vi "Robot Global Data.vi"() -> ()   [LabVIEW 2018]
doc: "This global VI can contain as many global variables as you need. Place a control on the panel, give it a good name. To read or write to it from a VI, drag the icon to the diagram of that VI. You can also drag from the project. Click on the node to change which global you access. You shouldn't have multiple locations writing to a global or it will cause a race-condition."
uses:
  <vilib>/Rock Robotics/WPI/DriverStation/WPI_DriverStationRobotMode2.ctl
panel:
  in  "Rottion_Control":dbl
  in  "Stage2_MotorControl 2":dbl
  in  "Stage1_MotorControl":dbl
  in  "manControl":bool
  out "DriverControllerButton12_input":bool
  in  "Stage 2_Lift PositionCurrent":string(combo)
  out "LIFT_EMERGENCY_STOP":bool
  in  "Lift Position_Desired":string(combo)
  out "DriverControllerButton11_input":bool
  out "DriveControllerButton10_input":bool
  out "DriveControllerButton9_input":bool
  out "DriveControllerButton8_input":bool
  out "DriveControllerButton7_input":bool
  out "DriveControllerButton6_input":bool
  out "DriveControllerButton5_input":bool
  out "DriveControllerButton4_input":bool
  out "DriveControllerButton3_input":bool
  out "DriveControllerButton2_input":bool
  out "DriveControllerButton1_input":bool
  out "DriveControllerRotation_AxisInput":dbl
  out "DriveControllerSide_AxisInput":dbl
  out "DriveControllerForwardBack_AxisInput":dbl
  out "DriveControllerThrottle_Input":dbl
  out "RobotDrive_Input":dbl
  out "RobotRotation_Input":dbl
  in  "Stage 1_LiftPositionCurrent":string(combo)
  in  "Robot Mode":T1
  # "Driver Controller Values"
  # "Axis"
  # "Buttons"
  # "This will probably be\na drives' station controlled \nbutton that the oporator will\npress if anything goes wrong"
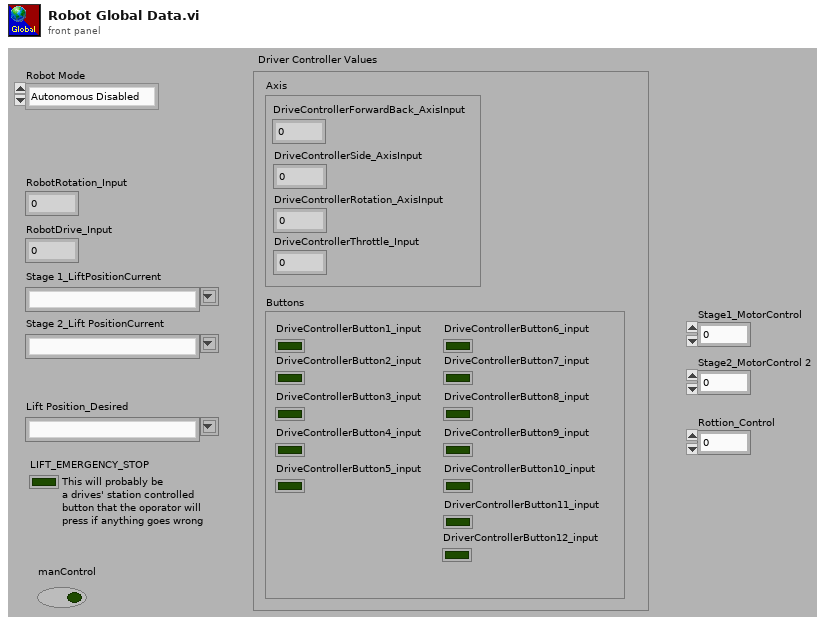
[diagram p1: front panel]
types:
  T1 = typedef "WPI_DriverStationRobotMode2.ctl" = enum16{"Autonomous Disabled", "Autonomous Enabled", "Teleop Disabled", "Teleop Enabled", "Disconnected", "Finish", "Test Disabled", "Test Enabled", "Emergency Stopped"}
diagram:
